vi "Get Value by Param Pattern.vi"(7 "Default Val":dbl, 8 "error in (no error)":errorcluster, 9 "Pattern":string, 10 "[Values]":variant[](array[variant]), 11 "[Params]":string[](array[string])) -> (0 "error out":errorcluster, 3 "[Values out]":dbl[](array[numeric]))   [LabVIEW 2018, in "RT - Analysis.lvlib"]
uses:
  RT - Analysis.lvlib
  <userlib>/_OpenG.lib/array/array.llb/Index 1D Array Elements (Variant)__ogtk.vi
panel:
  out "all lower case string":string[](array[string])
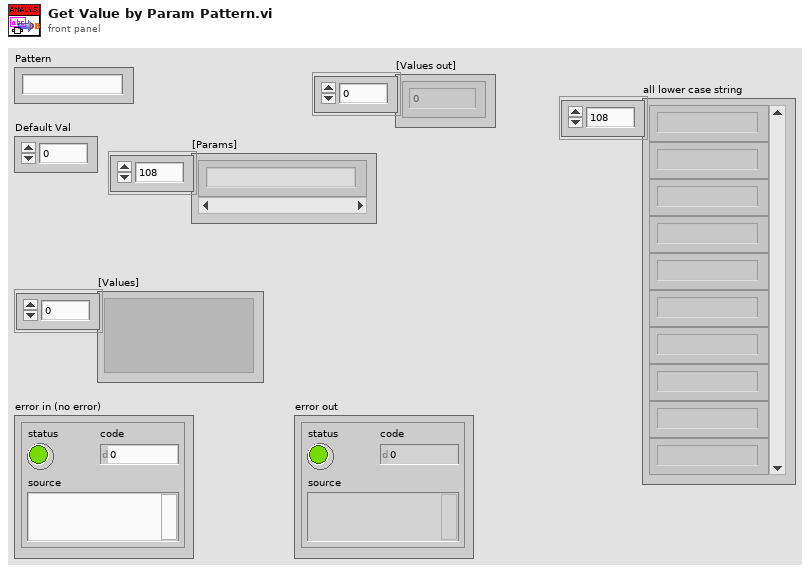
[diagram p1: front panel]
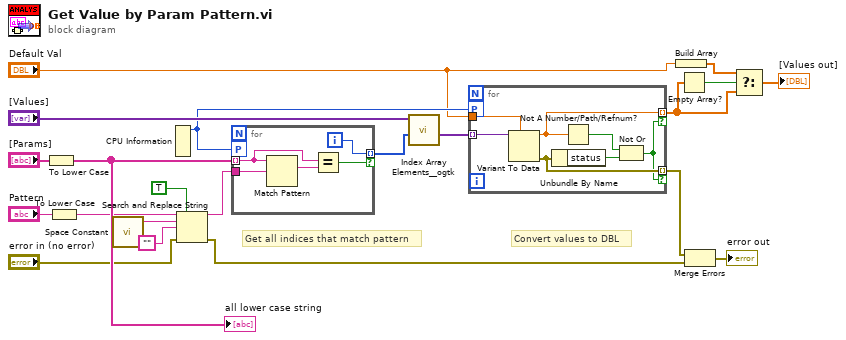
[diagram p0: block diagram]
diagram:
  # "Convert values to DBL"
  # "Get all indices that match pattern"
  n1 = To Lower Case(string="[Params]") -> (all lower case string=w14:string[])
  "all lower case string" <- w14
  n2 = To Lower Case(string="Pattern") -> (all lower case string=w13:string)
  n3 = call <vilib>:"Space Constant.vi"() -> ("String"=w11:string)
  n4 = CPU Information() -> (4:w7:i32)  [unwired: 3 out]
  n5 = Search and Replace String(replace all?=TRUE ("replace all? (F)"), input string=w13, search string=w11, replace string="", error in="error in (no error)") -> (result string=w12:string, error out=w8:errorcluster)  [unwired: 3 in, 2 out]
  n6 = for {
    tunnel: w14 -> [w22] mode=indexing
    tunnel: [w26] -> w18 mode=indexing if=w23
    tunnel: w12 -> [w25]
    workers-P: w7 -> [_]
    i -> [w26]
    n7 = Match Pattern(string=w22, regular expression=w25) -> (match substring=w24:string)  [unwired: 1 in, 3 out]
    n8 = Equal?(x=w22, y=w24) -> (x = y?=w23:bool)
  }
  n9 = call-poly <userlib>:"Index Array Elements__ogtk.vi"("indices"=w18, "array"="[Values]") -> ("elements"=w19:variant[])  [unwired: 9 in]
  n10 = for {
    tunnel: w19 -> [w33] mode=indexing
    tunnel: "Default Val" -> [w32]
    tunnel: [w30] -> w20 mode=indexing if=w27
    tunnel: [w31] -> w4 mode=indexing if=w27
    workers-P: w7 -> [_]
    n11 = Variant To Data(type=w32, Variant=w33) -> (data=w31:dbl, error out=w30:errorcluster)  [unwired: 1 in]
    n12 = Unbundle By Name(w30) -> ("status"=w28:bool)
    n13 = Not A Number/Path/Refnum?(number/path/refnum=w31) -> (NaN/Path/Refnum?=w29:bool)
    n14 = Not Or(1:w28, 2:w29) -> (0:w27:bool)
  }
  n15 = Build Array("Default Val") -> (w3:dbl[])
  n16 = Empty Array?(array=w4) -> (empty?=w6:bool)
  n17 = Merge Errors(w20, w8) -> (→"error out":errorcluster)
  n18 = Select(t=w3, s=w6, f=w4) -> (s? t:f=→"[Values out]":dbl[])
